vi "New Configuration to DSF Configuration Session v2.vi"(8 "error in":errorcluster, 11 "config data ref in":T1) -> (0 "error out":errorcluster, 3 "config data ref out":T1)   [LabVIEW 2017, in "DSF Configuration.lvlib" / "Configuration Session.lvclass"]
uses:
  Configuration Session.lvclass
  Config Data Ref.ctl
  DSF Configuration API/Private/Controls/Session/DSF Config Data.ctl
  DSF Configuration API/Private/Controls/DSF File Format/Internal.DSF Configuration.ctl
  DSF Configuration API/Public/Controls/DSF Version Info.ctl
  DSF Configuration API/Private/Controls/DSF File Format/Internal.DSF Plugin with ID.ctl
  DSF Configuration API/Private/Controls/DSF File Format/Internal.DSF Plugin Info.ctl
  DSF Configuration API/Public/Controls/DSF Timing Info.ctl
  DSF Configuration API/Private/Controls/DSF File Format/Internal.DSF Group with ID.ctl
  DSF Configuration API/Private/Controls/DSF File Format/Internal.DSF Group Info.ctl
  DSF Configuration API/Private/Controls/DSF File Format/Internal.DSF Transfer with ID.ctl
  DSF Configuration API/Private/Controls/DSF File Format/Internal.DSF Transfer Info.ctl
  DSF Configuration API/Private/Controls/DSF File Format/Internal.DSF Channel with ID.ctl
  DSF Configuration API/Private/Controls/DSF File Format/Internal.DSF Channel Info.ctl
  DSF Configuration API/Private/Controls/DSF File Format/Internal.DSF Settings with ID.ctl
  DSF Configuration API/Private/Controls/DSF File Format/Internal.DSF Settings Info.ctl
  DSF Configuration.lvlib
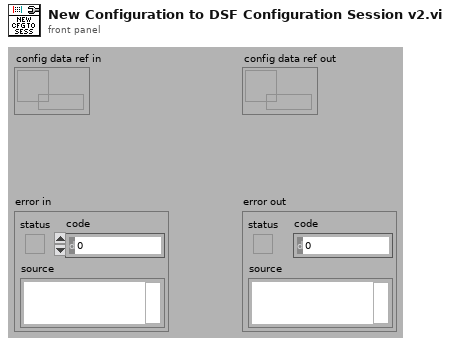
[diagram p1: front panel]
types:
  T1 = typedef "DSF Configuration.lvlib/Configuration Session.lvclass/Config Data Ref.ctl" = refnum<data-value>
  T2 = typedef "DSF Configuration.lvlib/DSF Version Info.ctl" = cluster{"major":u32, "minor":u32, "fix":u32, "build":string}
  T3 = typedef "DSF Configuration.lvlib/Configuration Session.lvclass/Internal.DSF Configuration.ctl" = cluster{"dsfversion":T2, "version":T2, "plugins":T4[], "groups":T7[], "transfers":T9[], "channels":T11[], "settings":T13[]}
  T4 = typedef "DSF Configuration.lvlib/Configuration Session.lvclass/Internal.DSF Plugin with ID.ctl" = cluster{"id":string, "values":T5}
  T5 = typedef "DSF Configuration.lvlib/Configuration Session.lvclass/Internal.DSF Plugin Info.ctl" = cluster{"type":string, "timing":T6, "group ids":string[], "settings id":string}
  T6 = typedef "DSF Configuration.lvlib/DSF Timing Info.ctl" = cluster{"priority":u64, "decimation":u64, "offset":u64}
  T7 = typedef "DSF Configuration.lvlib/Configuration Session.lvclass/Internal.DSF Group with ID.ctl" = cluster{"id":string, "values":T8}
  T8 = typedef "DSF Configuration.lvlib/Configuration Session.lvclass/Internal.DSF Group Info.ctl" = cluster{"direction":i32, "timing":T6, "transfer ids":string[], "settings id":string}
  T9 = typedef "DSF Configuration.lvlib/Configuration Session.lvclass/Internal.DSF Transfer with ID.ctl" = cluster{"id":string, "values":T10}
  T10 = typedef "DSF Configuration.lvlib/Configuration Session.lvclass/Internal.DSF Transfer Info.ctl" = cluster{"byte order":i32, "channel ids":string[], "settings id":string}
  T11 = typedef "DSF Configuration.lvlib/Configuration Session.lvclass/Internal.DSF Channel with ID.ctl" = cluster{"id":string, "values":T12}
  T12 = typedef "DSF Configuration.lvlib/Configuration Session.lvclass/Internal.DSF Channel Info.ctl" = cluster{"count":u64, "buffer offset":u64, "data type":i32, "settings id":string}
  T13 = typedef "DSF Configuration.lvlib/Configuration Session.lvclass/Internal.DSF Settings with ID.ctl" = cluster{"id":string, "values":T14}
  T14 = typedef "DSF Configuration.lvlib/Configuration Session.lvclass/Internal.DSF Settings Info.ctl" = cluster{"key":string, "value":string}[]
  T15 = typedef "DSF Configuration.lvlib/Configuration Session.lvclass/DSF Config Data.ctl" = cluster{"dsf configuration":T3, "path":path, "dirty":bool}
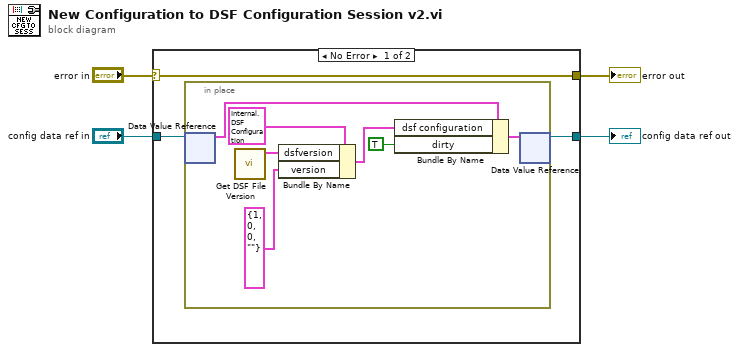
[diagram p0: block diagram]
diagram:
  n1 = case shown="No Error" "error in" {
    selector: "error in" -> [w7 w15]
    tunnel: [w7 w15] -> w4
    tunnel: [w5 w16] -> w1
    tunnel: "config data ref in" -> [w6 w16]
    frame No Error {
      n2 = in-place {
        n3 = in-place-dvr #1(w6) -> (w8:T15)  [unwired: 1 out]
        n4 = call "Get DSF File Version.vi"() -> ("dsf"=w11:T2)  [unwired: 11 in]
        n5 = Bundle By Name(cluster=T3 {"dsfversion"={"major"=0, "minor"=0, "fix"=0, "build"=""}, "version"={"major"=0, "minor"=0, "fix"=0, "build"=""}, "plugins"=[], "groups"=[], "transfers"=[], "channels"=[], "settings"=[]} ("dsf configuration"), "dsfversion"=w11, "version"=T2 {"major"=1, "minor"=0, "fix"=0, "build"=""}) -> (w12:T3)
        n6 = Bundle By Name(cluster=w8, "dsf configuration"=w12, "dirty"=TRUE) -> (w9:T15)
        n7 = in-place-dvr #1(w9) -> (w5:T1)  [unwired: 1 out]
      }
    }
    frame Error {
    }
  }
  "error out" <- w4
  "config data ref out" <- w1
